vi "FFT.vi"() -> ()   [LabVIEW 2024]
uses:
  <vilib>/Waveform/WDTOps.llb/WDT Get Waveform Subset DBL.vi
  <vilib>/measure/maspectr.llb/FFT Power Spectrum for N Chan.vi
  <vilib>/measure/NI_MAPro.lvlib
panel:
  in  "Data window":T1={"Start"=-0.01, "Length"=0.1, "Channel numbers"=[], "Cannel names (TDMS)"=["V"], "Group name"="p"} {"Length" format="%#_6ps"; "Start" format="%#_6ps"}
  out "Signal graph":waveform(dbl)[](graph)
  in  "Preserve prior FFT":bool
  out "FFT Graph":cluster{"f0":dbl, "df":dbl, "magnitude":dbl[]}[](graph)
  in  "Window":u32(ring)=1 items=["Rectangle"=0, "Hanning"=1, "Hamming"=2, "Blackman-Harris"=3, "Exact Blackman"=4, "Blackman"=5, "Flat Top"=6, "4 Term B-Harris "=7, "7 Term B-Harris"=8, "Low Sidelobe"=9, "Blackman Nuttall"=11, "Triangle"=30, "Bartlett-Hanning"=31, "Bohman"=32, "Parzen"=33, "Welch"=34, "Kaiser"=60, "Dolph-Chebyshev"=61, "Gaussian"=62]
  in  "Input file path":path
  # "OR (ASCII)"
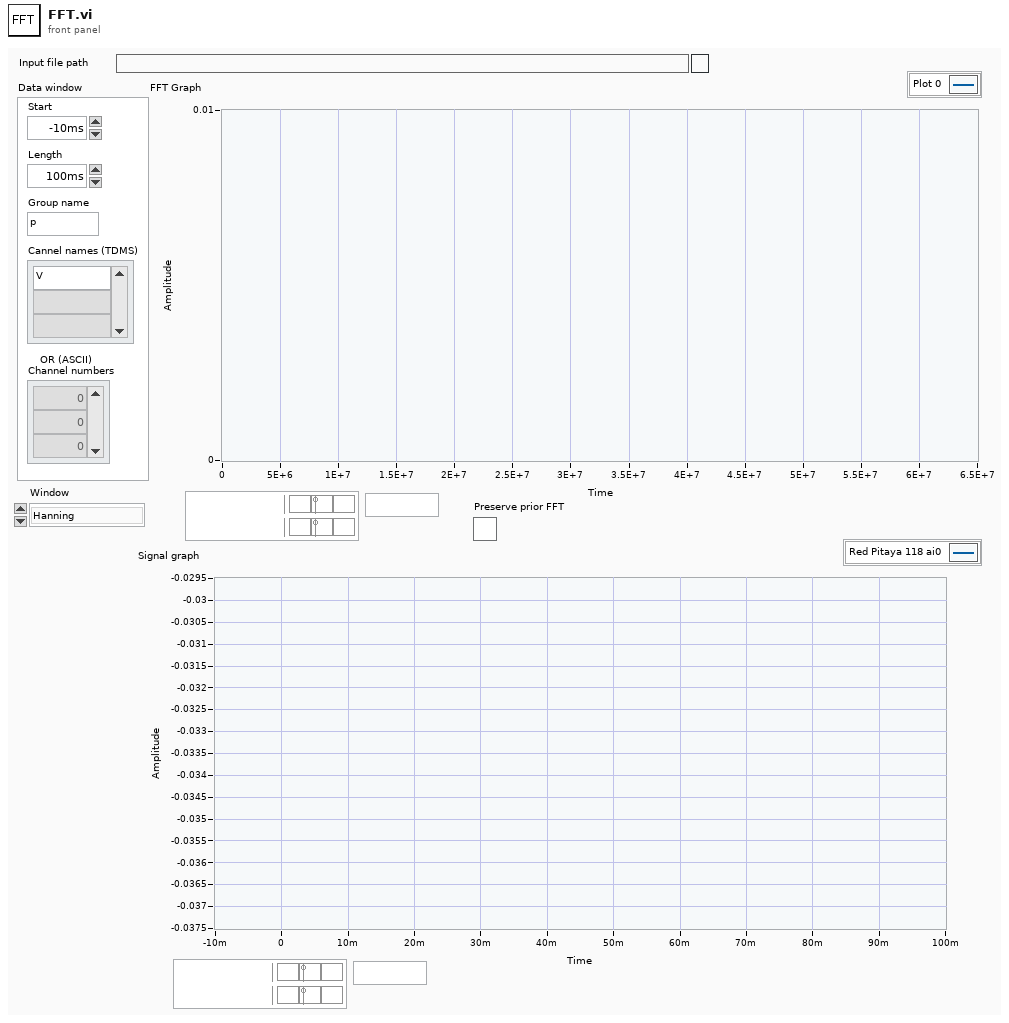
[diagram p1: front panel]
types:
  T1 = cluster{"Start":dbl, "Length":dbl, "Channel numbers":i64[], "Cannel names (TDMS)":string[], "Group name":string}
  T2 = enum16{"open", "open or create", "create or replace", "create", "open (read-only)"}
  T3 = enum16{"TDMS file", "Tektronics ISF", "BinF file", "ASCII File", "BinH File", "BinW File", "BINARY File"}
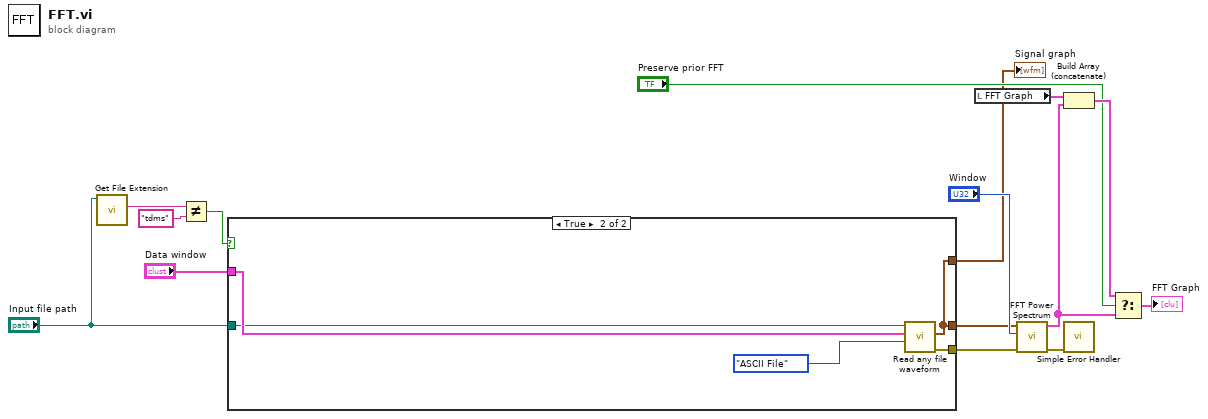
[diagram p0: block diagram]
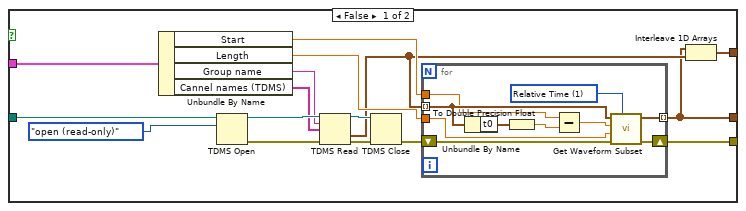
[diagram p2: hidden frame]
diagram:
  n1 = call <vilib>:"Get File Extension.vi"("file"="Input file path") -> ("lowercase file extension"=w5:string)  [unwired: 6 in, 4 out]
  n2 = Not Equal?(x=w5, y="tdms") -> (x != y?=w3:bool)
  n3 = case shown="True" w3 {
    tunnel: [w16 w46] -> w15
    tunnel: [w18 w43] -> w2
    tunnel: "Data window" -> [w28 w45]
    tunnel: "Input file path" -> [w31 w44]
    tunnel: [w17 w43] -> w1
    frame False {
      n4 = Unbundle By Name(w28) -> ("Start"=w21:dbl, "Length"=w20:dbl, "Group name"=w27:string, "Cannel names (TDMS)"=w26:string[])
      n5 = TDMS Open(10:T2."open (read-only)" ("operation (0:open)"), 11:w31) -> (0:w25:errorcluster, 3:w29:refnum<k34>)  [unwired: 5 in]
      n6 = TDMS Read(0:w29, 5:w27, 7:w26, 11:w25) -> (4:w23:refnum<k34>, 10:w19:waveform(dbl)[], 15:w24:errorcluster)  [unwired: 4 in, 3 out]
      n7 = TDMS Close(8:w24, 11:w23) -> (0:w22:errorcluster)  [unwired: 1 out]
      n8 = for {
        tunnel: w19 -> [w38] mode=indexing
        shift-right: [w40] -> w16
        shift-left: w22 -> [w41]
        tunnel: w21 -> [w35]
        tunnel: w20 -> [w33]
        tunnel: [w32] -> w18 mode=indexing
        w39 = u16 1 items=["Samples", "Relative Time"] ("start/duration format")
        n9 = Unbundle By Name(w38) -> ("t0"=w37:timestamp)
        n10 = To Double Precision Float(number=w37) -> (double precision float=w36:dbl)
        n11 = Subtract(x=w35, y=w36) -> (x-y=w34:dbl)
        n12 = call-poly <vilib>:"Get Waveform Subset.vi"("start/duration format"=w39, "error in (no error)"=w41, "duration"=w33, "start samples/time"=w34, "waveform in"=w38) -> ("error out"=w40:errorcluster, "waveform out"=w32:waveform(dbl))  [unwired: 1 in, 2 out]
      }
      n13 = Interleave 1D Arrays(w18, w19) -> (w17:waveform(dbl)[])
    }
    frame True {
      n14 = call "Read any file waveform.vi"("Data File Type"=T3."ASCII File", "Data window"=w45, "Input file path"=w44) -> ("error out"=w46:errorcluster, "Data out"=w43:waveform(dbl)[])  [unwired: 4 in, 3 out]
    }
  }
  "Signal graph" <- w1
  n15 = local read "FFT Graph"() -> (w13:cluster{"f0":dbl, "df":dbl, "magnitude":dbl[]}[])
  n16 = call-poly <vilib>:"FFT Power Spectrum.vi"("error in (no error)"=w15, "window"="Window", "time signals"=w2) -> ("error out"=w7:errorcluster, "power spectra"=w11:cluster{"f0":dbl, "df":dbl, "magnitude":dbl[]}[])  [unwired: 3 in, 4 out]
  n17 = Build Array (concatenate)(w13, w11) -> (w12:cluster{"f0":dbl, "df":dbl, "magnitude":dbl[]}[])
  n18 = call <vilib>:"Simple Error Handler.vi"("error in (no error)"=w7) -> ()  [unwired: 4 in, 5 out]
  n19 = Select(t=w12, s="Preserve prior FFT", f=w11) -> (s? t:f=→"FFT Graph":cluster{"f0":dbl, "df":dbl, "magnitude":dbl[]}[])
